vi "GOLPI full test.vi"() -> ()   [LabVIEW 2020, in "GOLPI library.lvlib"]
doc: "Makes test of all routines in GOLPI library. Good for testing changes in GOLPI library or testing compatibility with new versions of GNU Octave."
uses:
  GOLPI library.lvlib
  Type Definitions/Transfer Mode.ctl
  Type Definitions/Custom Error Codes Enum Type Def.vi
  Set Variable - polymorph parts/Set Double.vi
  Get Variable - polymorph parts/Get Double.vi
  Set Variable - polymorph parts/Set Double Complex.vi
  Get Variable - polymorph parts/Get Double Complex.vi
  Set Variable - polymorph parts/Set 2D Array Double.vi
  Get Variable - polymorph parts/Get 2D Array Double.vi
  Set Variable - polymorph parts/Set 2D Array Double Complex.vi
  Get Variable - polymorph parts/Get 2D Array Double Complex.vi
  Set Variable - polymorph parts/Set String.vi
  Get Variable - polymorph parts/Get String.vi
  Set Variable - polymorph parts/Set 1D Array String.vi
  Get Variable - polymorph parts/Get 1D Array String.vi
panel:
  out "file (write)":dbl format="%#_3p"
  out "pipe (write)":dbl format="%#_3p"
  out "console (write)":dbl format="%#_3p"
  out "pipe":dbl format="%#_3p"
  out "bitstream":dbl format="%#_3p"
  out "State":string
  in  "skip read to ...\n tests?":bool
  out "mode":T1
  in  "Matlab\nmode":bool
  out "file":dbl format="%#_3p"
  out "console":dbl format="%#_3p"
  in  "wait for exit\n(press this again to exit)":bool
  in  "hide window":bool
  out "now running test no:":i32
  out "all tests result":bool
  out "test results":T2(array[cluster])
  in  "do tests with large\nrandom datasets?":bool
  out "GNU Octave version":string
  out "exit code":i32
  out "error out":errorcluster
  in  "Octave binary directory":path=path "C:/Octave/Octave-4.2.2/bin/octave-cli.exe"
  in  "Working directory":path=path "C:/work"
  # "Runs various tests and checks all parts of GOLPI library.\nSelecting 'do tests with large random datasets' cause\nrunning of time consuming tests.\nIf all tests are OK, GOLPI is fully working with selected\nGNU Octave binary.\nIF WORKING DIRECTORY IS NOT WRITEABLE (C:\\ in Win7+), tests will fail also."
  # "Time consumed reading/writting large random matrix (s) using:"
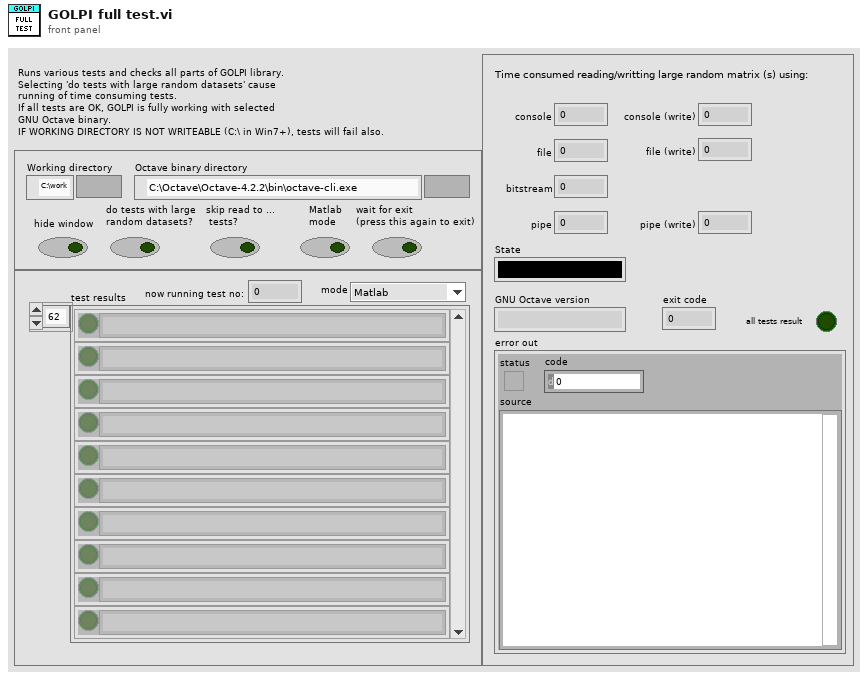
[diagram p1: front panel]
types:
  T1 = typedef "GOLPI library.lvlib/Transfer Mode.ctl" = enum16{"Matlab", "stdio", "temp file", "bitstream", "pipe"}
  T2 = cluster{"test result":bool, "variable name":string}[]
  T3 = typedef "GOLPI library.lvlib/GOLPI reference Type Def.ctl" = cluster{"pipe handle":T4, "fast read timeout [ms]":u32, "fast read settle time [ms]":u32, "fast read to multiple [ms]":u32, "max elements per input line":u32, "slow read timeout [ms]":u32, "stdin double format specifier":string, "max elements per stdout output column":u32, "console mode bitstream":bool, "bitstream first read timeout [ms]":u32, "bitstream read timeout [ms]":u32, "struct transfer possible":bool, "matlab mode":bool, "var pipe write timeout [ms]":u32, "variable pipe mode":bool, "variable pipe buffer size [Bytes]":u32, "variable pipe block size [Bytes]":u32}
  T4 = typedef "LV Process library.lvlib/Pipe Handle.ctl" = cluster{"lv_proc.dll file path":path, "process instance handle":u32[], "debug mode":bool, "debug data":cluster{"time":timestamp, "stdin":bool, "data":string}[]}
  T5 = typedef "GOLPI library.lvlib/Custom Error Codes Enum Type Def.vi" = enum16{"no error", "00 working directory PAR1 missing", "01 octave binary PAR1 missing", "02 octave report error PAR1", "03 empty output last cmd PAR1", "04 missing temporary file PAR1", "05 pwd PAR 1 not exist", "06 oct package not installed", "07 octave default binary missing", "10 var PAR1 not string, vect", "11 var PAR1 not num, scal, ~compl", "12 var PAR1 not num, scal, compl", "13 var PAR1 not num, vect, ~compl", "14 var PAR1 not num, vect, compl", "15 var PAR1 not num, mat, ~compl", "16 var PAR1 not num, mat, ~compl", "30 read timeout", "60 bitstream transport failed", "61 bitstream decode error PAR1", "62 bitstream cannot be set", "70 struct transfer not possible", "80 struct: cluster elem. PAR1 not implem.", "81 struct: structure field PAR1 not implem.", "82 struct: size mismatch of PAR1", "83 struct: type mismatch of PAR1", "98 internal error", "99 not finished", "90 Not supported in Matlab mode", "91 Matlab variable transfer error", "92 Matlab Script Error", "100 Variable Pipe Mode cannot be set"}
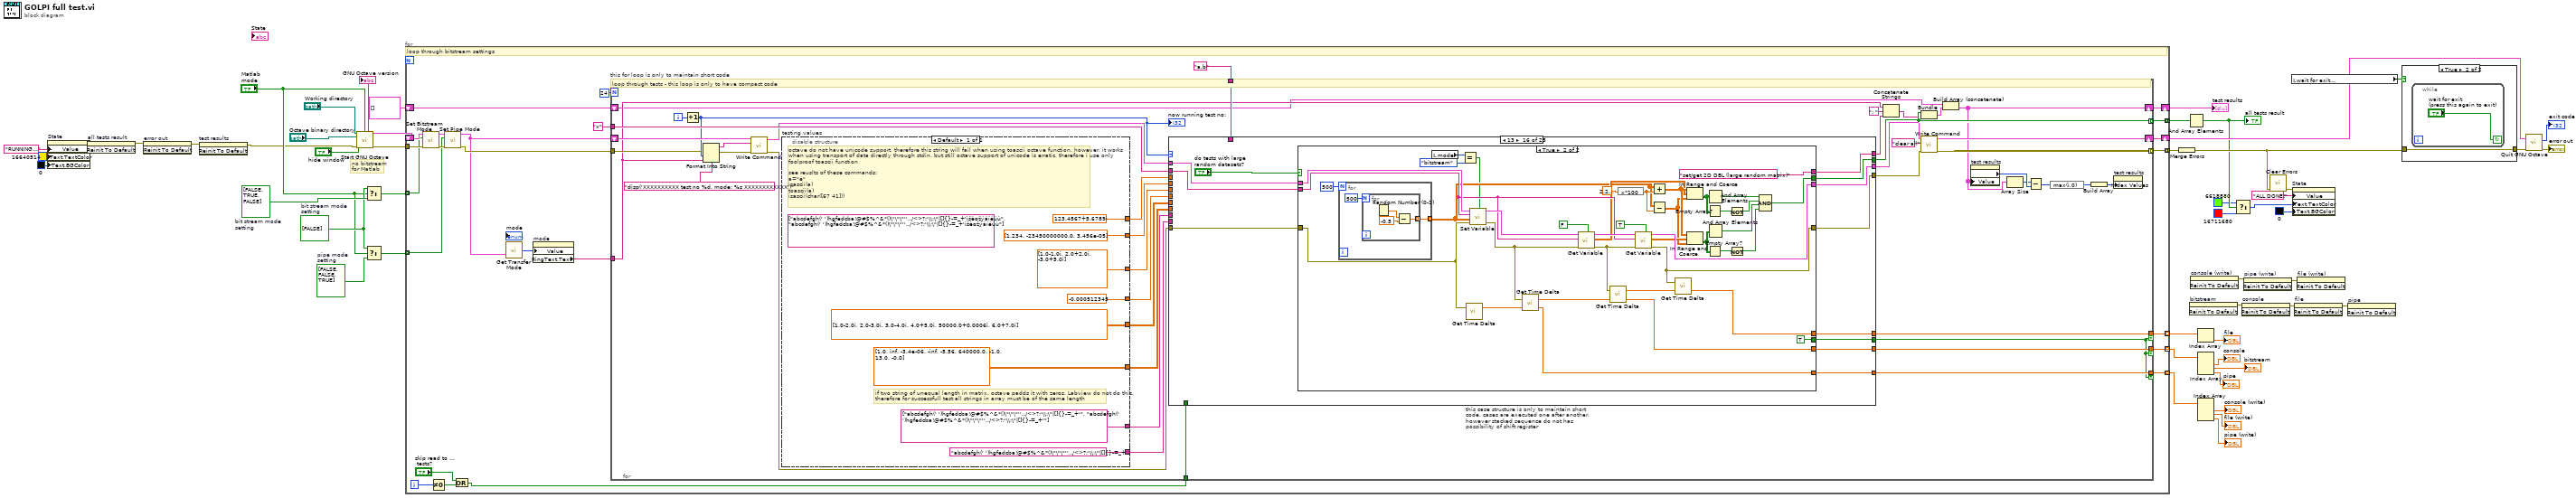
[diagram p0: block diagram]
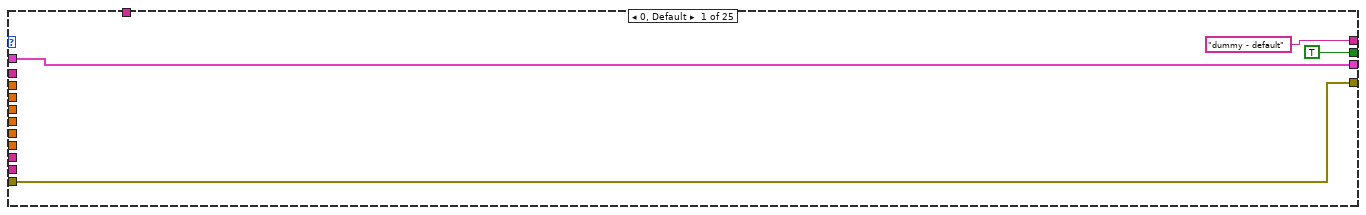
[diagram p3: hidden frame]
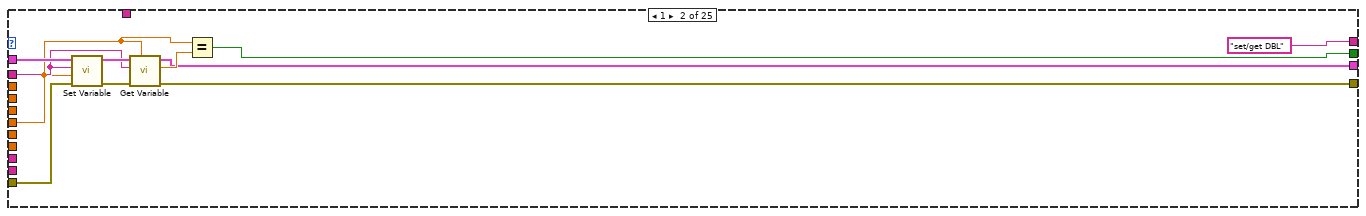
[diagram p4: hidden frame]
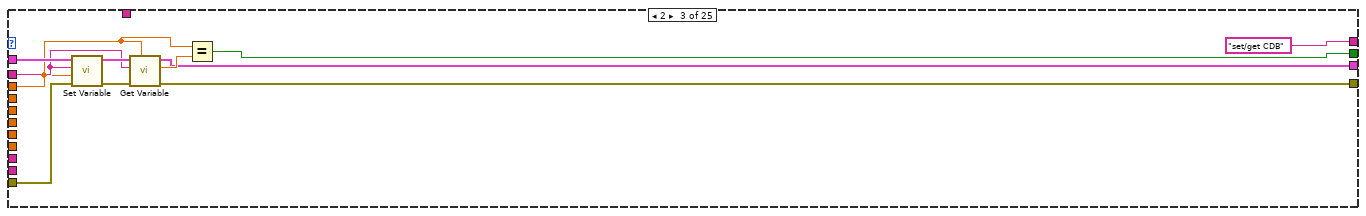
[diagram p5: hidden frame]
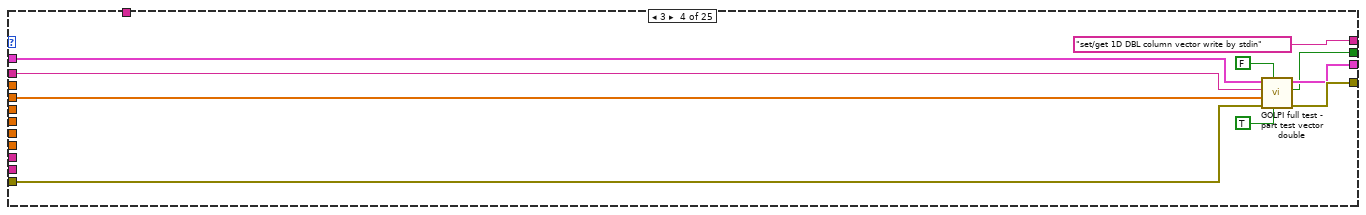
[diagram p6: hidden frame]
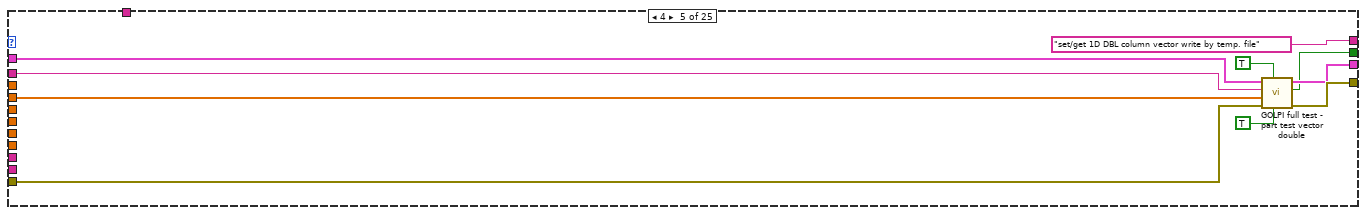
[diagram p7: hidden frame]
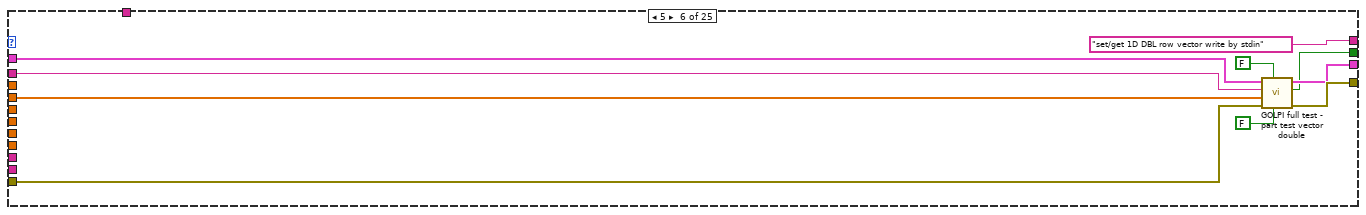
[diagram p8: hidden frame]
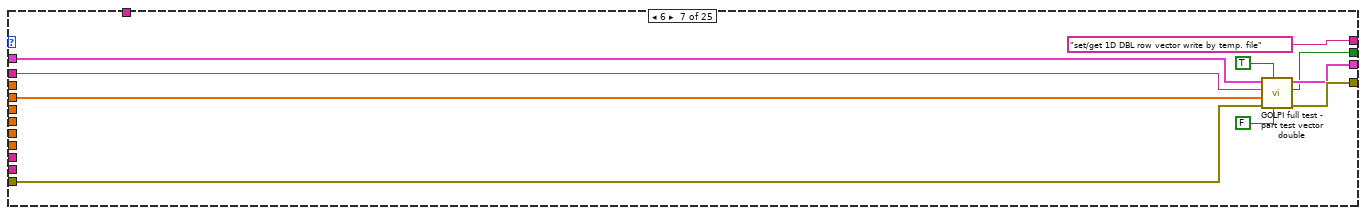
[diagram p9: hidden frame]
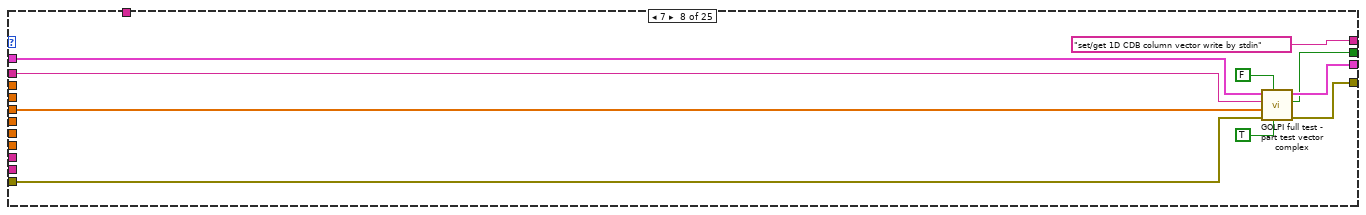
[diagram p10: hidden frame]
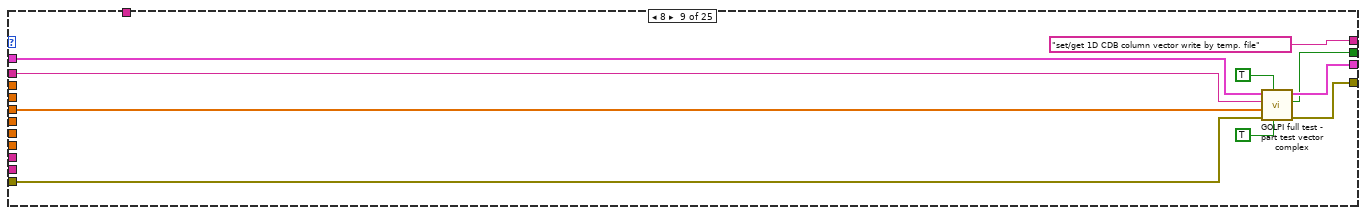
[diagram p11: hidden frame]
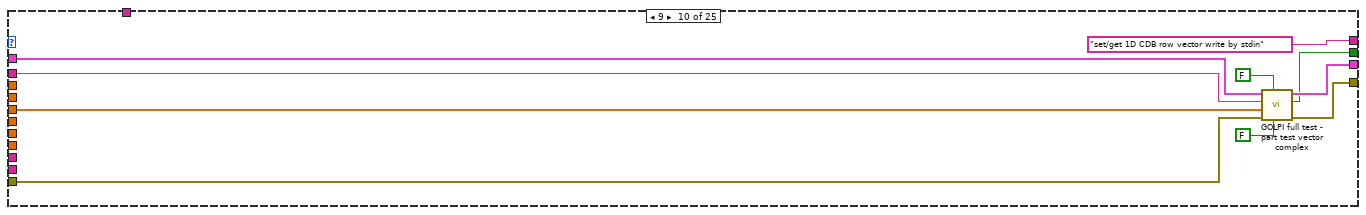
[diagram p12: hidden frame]
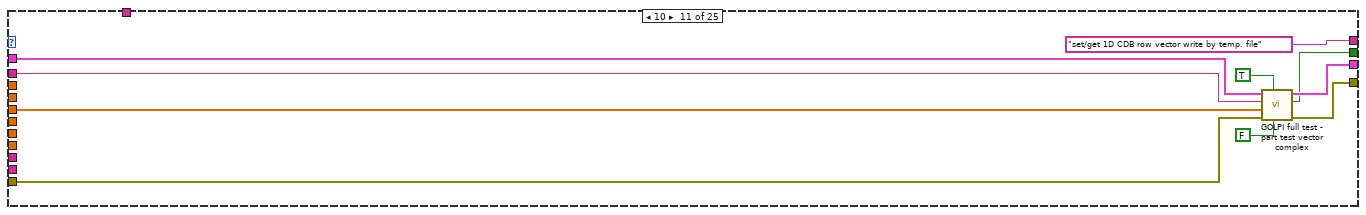
[diagram p13: hidden frame]
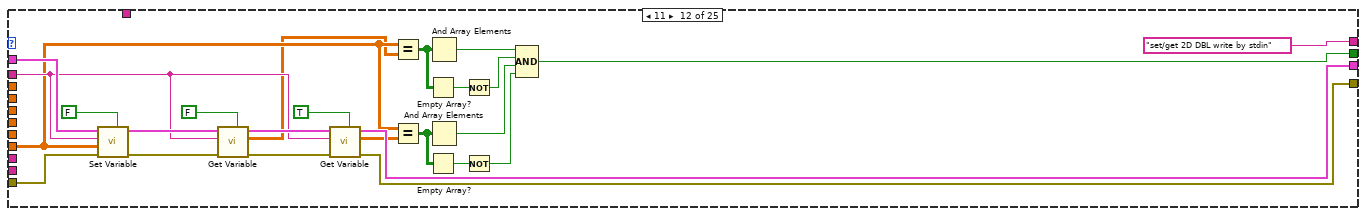
[diagram p14: hidden frame]
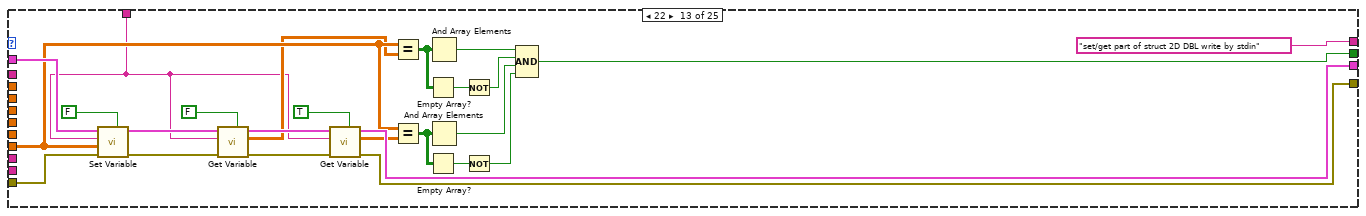
[diagram p15: hidden frame]
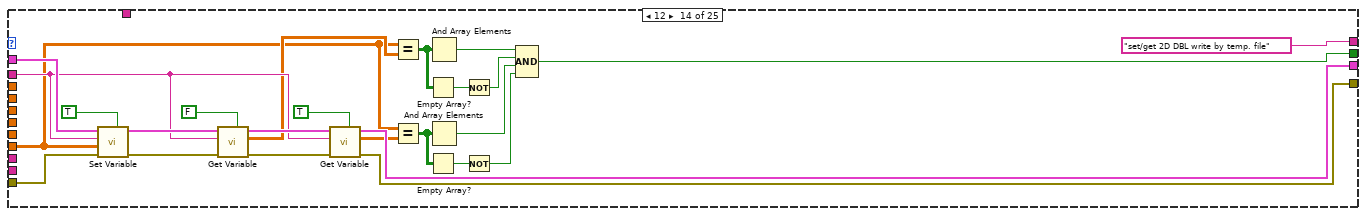
[diagram p16: hidden frame]
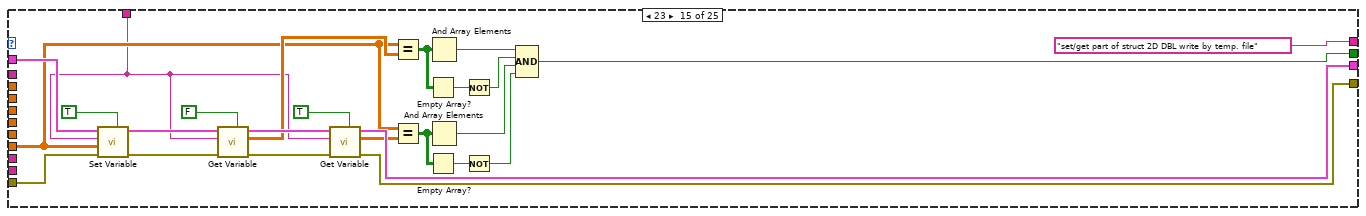
[diagram p17: hidden frame]
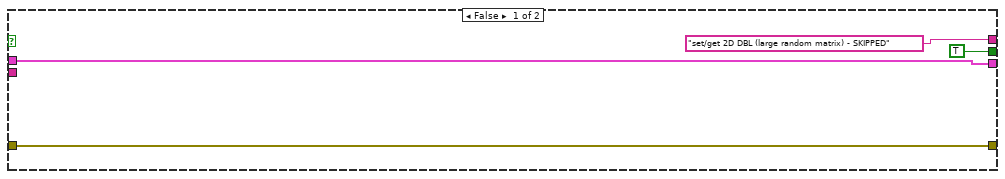
[diagram p18: hidden frame]
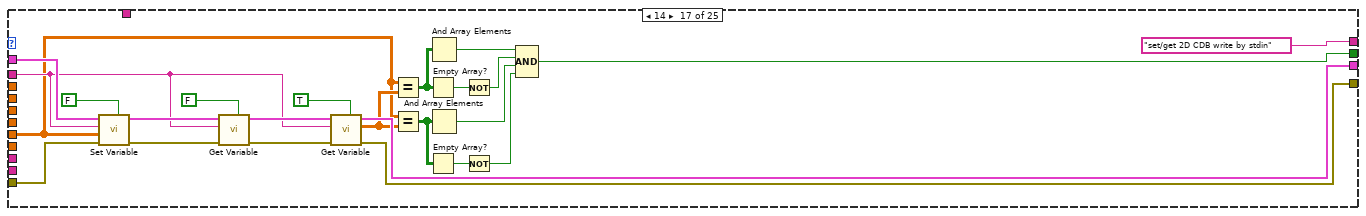
[diagram p19: hidden frame]
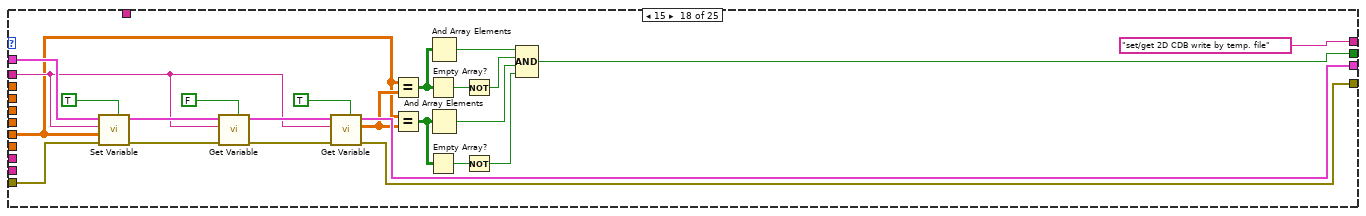
[diagram p20: hidden frame]
diagram:
  w38 = bool[] [FALSE, FALSE, TRUE]  # pipe mode setting
  w39 = bool[] [FALSE]  # bit stream mode setting
  w41 = bool[] [FALSE, TRUE, FALSE]  # bit stream mode setting
  # "no bitstream\nfor Matlab"
  n1 = property on="State" class="Str"("Value"="RUNNING..." ("State"), "Text.TextColor"=u32 16640514 ("Text.Text Colors:Text Color"), "Text.BGColor"=u32 0 ("Text.Text Colors:BG Color")) -> (error out=w27:errorcluster)  [unwired: 2 in, 1 out]
  n2 = invoke on="all tests result" class="Bool (strict)" method="Reinit To Default"(error in=w27) -> (error out=w28:errorcluster)  [unwired: 2 in, 2 out]
  n3 = invoke on="error out" class="Clust (strict)" method="Reinit To Default"(error in=w28) -> (error out=w36:errorcluster)  [unwired: 2 in, 2 out]
  n4 = invoke on="test results" class="Arr (strict)" method="Reinit To Default"(error in=w36) -> (error out=w35:errorcluster)  [unwired: 2 in, 2 out]
  n5 = call "Start GNU Octave.vi"("working dir (user home)"="Working directory", "Matlab script mode (F)"="Matlab\nmode", "octave binary file or dir (autofind)"="Octave binary directory", "hide debug console (T)"="hide window", "error in"=w35) -> ("GNU Octave version"=→"GNU Octave version":string, "GOLPI ref. out"=w45:T3, "error out"=w49:errorcluster)  [unwired: 7 in, 1 out]
  n6 = Select(t=w39, s="Matlab\nmode", f=w41) -> (s? t:f=w42:bool[])
  n7 = Select(t=w39, s="Matlab\nmode", f=w38) -> (s? t:f=w40:bool[])
  n8 = for {
    tunnel: [w73] -> w48 mode=concatenating
    shift-right: [w75] -> w43
    shift-left: w45 -> [w69]
    tunnel: w42 -> [w68] mode=indexing
    tunnel: w49 -> [w70]
    tunnel: [w71] -> w44 mode=concatenating
    tunnel: w40 -> [w64] mode=indexing
    shift-right: [w56] -> w30
    shift-left: cluster{"test result":bool, string}[] [] -> [w55]
    tunnel: [w54] -> w15 mode=indexing
    tunnel: [w53] -> w13 mode=indexing
    tunnel: [w52] -> w6 mode=indexing
    i -> [w60]
    # "loop through bitstream settings"
    n9 = call "Set Bitstream Mode.vi"("error in"=w70, "Bitstream mode (F)"=w68, "GOLPI ref. in"=w69) -> ("error out"=w67:errorcluster, "GOLPI ref. out"=w66:T3)  [unwired: 7 in]
    n10 = Not Equal To 0?(x=w60) -> (x != 0?=w59:bool)
    n11 = call "Set Pipe Mode.vi"("error in"=w67, "Variable Pipe Mode? (F)"=w64, "GOLPI ref. in"=w66) -> ("error out"=w65:errorcluster, "GOLPI ref. out"=w63:T3)  [unwired: 7 in]
    n12 = Compound Arithmetic op=OR("skip read to ...\n tests?", w59) -> (w57:bool)
    n13 = call "Get Transfer Mode.vi"("GOLPI ref."=w63) -> ("mode"=w62:T1)  [unwired: 1 in]
    n14 = property on="mode" class="Enum (strict)"("Value"=w62) -> ("RingText.Text"=w61:string)  [unwired: 2 in, 2 out]
    n15 = for "this for loop is only to maintain short code" {
      N: 24 -> [_]
      tunnel: "x" ("variable name") -> [w118]
      shift-right: [w114] -> w75
      shift-left: w63 -> [w100]
      tunnel: [w116] -> w73 mode=indexing
      tunnel: "a.b" ("variable name") -> [w102]
      tunnel: w65 -> [w96]
      tunnel: [w112] -> w71 mode=indexing
      tunnel: w61 -> [w91]
      tunnel: w57 -> [w89]
      shift-right: [w81] -> w56
      shift-left: w55 -> [w87]
      tunnel: [w80] -> w54 if=w77
      tunnel: [w79] -> w53 if=w77
      tunnel: [w78] -> w52 if=w77
      i -> [w117]
      # "loop through tests - this loop is only to have compact code"
      n16 = Increment(x=w117) -> (x+1=w97:i32)
      "now running test no:" <- w97
      n17 = Format Into String(format string="disp('XXXXXXXXXX test no %d, mode: %s XXXXXXXXXXXX')", error in=w96, w97, w91) -> (resulting string=w94:string, error out=w95:errorcluster)  [unwired: 1 in]
      n18 = call "Write Command.vi"("error in"=w95, "command"=w94, "GOLPI ref. in"=w100) -> ("error out"=w101:errorcluster, "GOLPI ref. out"=w99:T3)  [unwired: 7 in]
      n19 = disable-structure "testing values" shown="Default" {
        disable-tunnel: [-0.000512345 ("value")] -> w110
        disable-tunnel: [dbl[] [1.234, -23450000000.0, 3.456e-05] ("value")] -> w109
        disable-tunnel: [cdb[] [1.0-1.0i, 2.0+2.0i, -3.0+5.0i] ("value")] -> w108
        disable-tunnel: [dbl[][] [[1.0, inf, -3.4e-06], [-inf, -5.56, 640000.0], [-1.0, 13.0, -0.0]] ("value")] -> w107
        disable-tunnel: [cdb[][] [[1.0-2.0i, 2.0-3.0i, 3.0-4.0i], [4.0+5.0i, 50000.0+0.0006i, 6.0+7.0i]] ("value")] -> w106
        disable-tunnel: ["abcdefgh(' ')hgfedcba!@#$%^&*()\"\"\"'',./<>?;'\\:\"|[]{}-=_+'" ("value")] -> w105
        disable-tunnel: [string[] ["abcdefgh(' ')hgfedcba!@#$%^&*()\"\"\"'',./<>?;'\\:\"|[]{}-=_+'", "abcdefgh(' ')hgfedcba!@#$%^&*()\"\"\"'',./<>?;'\\:\"|[]{}-=_+'"]] -> w104
        disable-tunnel: [cdb 123.4567+5.6789i ("value")] -> w103
        frame Enabled {
          (unwired) string[] ["abcdefgh(' ')hgfedcba!@#$%^&*()\"\"\"'',./<>?;'\\:\"|[]{}-=_+'ìšèøžýáíéúù", "abcdefgh(' ')hgfedcba!@#$%^&*()\"\"\"'',./<>?;'\\:\"|[]{}-=_+'ìšèøžýáíéúù"]
          # "octave do not have unicode support, therefore this string will fail when using toascii octave function. however, it works\nwhen using transport of data directly through stdin. but still octave support of unicode is erratic, therefore i use only\nfoolproof toascii function\n\nsee reuslts of these commands:\na=\"é\"\nisascii(a)\ntoascii(a)\nisascii(char([67 41]))"
          # "if two string of unequal length in matrix, octave padds it with zeros. Labview do not do this.\ntherefore for successfull test all strings in array must be of the same length"
        }
      }
      n20 = case "this case structure is only to maintain short code. cases are executed one after another. however stacked sequence do not has possibility of shift register" shown="13" w97 {
        tunnel: w99 -> [w129 w138 w145 w158 w168 w180 w190 w202 w212 w219 w229 w253 w278 w303 w328 w340 w415 w439 w457 w476 w501 w526 w535 w565 w600]
        tunnel: w101 -> [w130 w137 w146 w161 w171 w182 w192 w199 w209 w222 w232 w254 w279 w304 w329 w341 w416 w440 w458 w477 w502 w527 w534 w564 w601]
        tunnel: [w130 w136 w147 w160 w170 w179 w189 w200 w210 w221 w231 w256 w281 w306 w331 w343 w414 w438 w450 w467 w489 w510 w531 w560 w593] -> w113
        tunnel: [w129 w135 w148 w159 w169 w178 w188 w201 w211 w220 w230 w255 w280 w305 w330 w342 w413 w437 w451 w465 w488 w512 w533 w562 w599] -> w115
        tunnel: w118 -> [_ w134 w144 w157 w167 w181 w191 w198 w208 w218 w228 w240 _ w290 _ w339 w395 w419 w448 w461 w487 w509 _ _ _]
        tunnel: [TRUE w133 w149 w154 w164 w177 w187 w196 w206 w215 w225 w257 w282 w307 w332 w344 w412 w436 w442 w463 w492 w517 w532 w561 w591] -> w116
        tunnel: ["dummy - default" ("variable name") "set/get DBL" ("variable name") "set/get CDB" ("variable name") "set/get 1D DBL column vector write by stdin" ("variable name") "set/get 1D DBL column vector write by temp. file" ("variable name") "set/get 1D DBL row vector write by stdin" ("variable name") "set/get 1D DBL row vector write by temp. file" ("variable name") "set/get 1D CDB column vector write by stdin" ("variable name") "set/get 1D CDB column vector write by temp. file" ("variable name") "set/get 1D CDB row vector write by stdin" ("variable name") "set/get 1D CDB row vector write by temp. file" ("variable name") "set/get 2D DBL write by stdin" ("variable name") "set/get part of struct 2D DBL write by stdin" ("variable name") "set/get 2D DBL write by temp. file" ("variable name") "set/get part of struct 2D DBL write by temp. file" ("variable name") w338 "set/get 2D CDB write by stdin" ("variable name") "set/get 2D CDB write by temp. file" ("variable name") "set/get STR write by stdin" ("variable name") "set/get STR write by temp. file" ("variable name") "set/get 1D STR write by stdin" ("variable name") "set/get 1D STR write by temp. file" ("variable name") w530 w563 "read struct" ("variable name")] -> w93
        tunnel: w110 -> [_ w131 _ _ _ _ _ _ _ _ _ _ _ _ _ _ _ _ _ _ _ _ _ _ _]
        tunnel: w103 -> [_ _ w142 _ _ _ _ _ _ _ _ _ _ _ _ _ _ _ _ _ _ _ _ _ _]
        tunnel: w109 -> [_ _ _ w153 w163 w173 w183 _ _ _ _ _ _ _ _ _ _ _ _ _ _ _ _ _ _]
        tunnel: w108 -> [_ _ _ _ _ _ _ w193 w203 w213 w223 _ _ _ _ _ _ _ _ _ _ _ _ _ _]
        tunnel: w107 -> [_ _ _ _ _ _ _ _ _ _ _ w235 w261 w283 w309 _ _ _ _ _ _ _ _ _ _]
        tunnel: w106 -> [_ _ _ _ _ _ _ _ _ _ _ _ _ _ _ _ w393 w417 _ _ _ _ _ _ _]
        tunnel: w105 -> [_ _ _ _ _ _ _ _ _ _ _ _ _ _ _ _ _ _ w441 w460 _ _ _ _ _]
        tunnel: w104 -> [_ _ _ _ _ _ _ _ _ _ _ _ _ _ _ _ _ _ _ _ w479 w504 _ _ _]
        tunnel: w102 -> [_ _ _ _ _ _ _ _ _ _ _ _ w258 _ w308 _ _ _ _ _ _ _ _ _ _]
        tunnel: w89 -> [_ _ _ _ _ _ _ _ _ _ _ _ _ _ _ _ _ _ _ _ _ _ w529 w559 _]
        tunnel: [_ _ _ _ _ _ _ _ _ _ _ _ _ _ _ w336 _ _ _ _ _ _ _ _ _] -> w80
        tunnel: [_ _ _ _ _ _ _ _ _ _ _ _ _ _ _ w335 _ _ _ _ _ _ _ _ _] -> w79
        tunnel: [_ _ _ _ _ _ _ _ _ _ _ _ _ _ _ w334 _ _ _ _ _ _ _ _ _] -> w77
        tunnel: [_ _ _ _ _ _ _ _ _ _ _ _ _ _ _ w333 _ _ _ _ _ _ _ _ _] -> w78
        frame 0, Default {
        }
        frame 1 {
          n21 = call-poly "Set Variable.vi"("error in"=w137, "value"=w131, "variable name"=w134, "GOLPI ref. in"=w138) -> ("error out"=w140:errorcluster, "GOLPI ref. out"=w141:T3)  [unwired: 6 in]
          n22 = call-poly "Get Variable.vi"("data type of variable"=w131, "error in"=w140, "variable name"=w134, "GOLPI ref. in"=w141) -> ("error out"=w136:errorcluster, "value"=w139:dbl, "GOLPI ref. out"=w135:T3)  [unwired: 5 in]
          n23 = Equal?(x=w131, y=w139) -> (x = y?=w133:bool)
        }
        frame 2 {
          n24 = call-poly "Set Variable.vi"("error in"=w146, "value"=w142, "variable name"=w144, "GOLPI ref. in"=w145) -> ("error out"=w151:errorcluster, "GOLPI ref. out"=w150:T3)  [unwired: 6 in]
          n25 = call-poly "Get Variable.vi"("data type of variable"=w142, "error in"=w151, "variable name"=w144, "GOLPI ref. in"=w150) -> ("error out"=w147:errorcluster, "value"=w152:cdb, "GOLPI ref. out"=w148:T3)  [unwired: 5 in]
          n26 = Equal?(x=w142, y=w152) -> (x = y?=w149:bool)
        }
        frame 3 {
          n27 = call "GOLPI full test - part test vector double.vi"("column vector?"=TRUE, "set: use temporary file?"=FALSE, "error in (no error)"=w161, "test value"=w153, "variable name in"=w157, "GOLPI ref. in"=w158) -> ("error out"=w160:errorcluster, "test result"=w154:bool, "GOLPI ref. out"=w159:T3)  [unwired: 3 in]
        }
        frame 4 {
          n28 = call "GOLPI full test - part test vector double.vi"("column vector?"=TRUE, "set: use temporary file?"=TRUE, "error in (no error)"=w171, "test value"=w163, "variable name in"=w167, "GOLPI ref. in"=w168) -> ("error out"=w170:errorcluster, "test result"=w164:bool, "GOLPI ref. out"=w169:T3)  [unwired: 3 in]
        }
        frame 5 {
          n29 = call "GOLPI full test - part test vector double.vi"("column vector?"=FALSE, "set: use temporary file?"=FALSE, "error in (no error)"=w182, "test value"=w173, "variable name in"=w181, "GOLPI ref. in"=w180) -> ("error out"=w179:errorcluster, "test result"=w177:bool, "GOLPI ref. out"=w178:T3)  [unwired: 3 in]
        }
        frame 6 {
          n30 = call "GOLPI full test - part test vector double.vi"("column vector?"=FALSE, "set: use temporary file?"=TRUE, "error in (no error)"=w192, "test value"=w183, "variable name in"=w191, "GOLPI ref. in"=w190) -> ("error out"=w189:errorcluster, "test result"=w187:bool, "GOLPI ref. out"=w188:T3)  [unwired: 3 in]
        }
        frame 7 {
          n31 = call "GOLPI full test - part test vector complex.vi"("column vector?"=TRUE, "set: use temporary file?"=FALSE, "error in (no error)"=w199, "test value"=w193, "variable name in"=w198, "GOLPI ref. in"=w202) -> ("error out"=w200:errorcluster, "test result"=w196:bool, "GOLPI ref. out"=w201:T3)  [unwired: 3 in]
        }
        frame 8 {
          n32 = call "GOLPI full test - part test vector complex.vi"("column vector?"=TRUE, "set: use temporary file?"=TRUE, "error in (no error)"=w209, "test value"=w203, "variable name in"=w208, "GOLPI ref. in"=w212) -> ("error out"=w210:errorcluster, "test result"=w206:bool, "GOLPI ref. out"=w211:T3)  [unwired: 3 in]
        }
        frame 9 {
          n33 = call "GOLPI full test - part test vector complex.vi"("column vector?"=FALSE, "set: use temporary file?"=FALSE, "error in (no error)"=w222, "test value"=w213, "variable name in"=w218, "GOLPI ref. in"=w219) -> ("error out"=w221:errorcluster, "test result"=w215:bool, "GOLPI ref. out"=w220:T3)  [unwired: 3 in]
        }
        frame 10 {
          n34 = call "GOLPI full test - part test vector complex.vi"("column vector?"=FALSE, "set: use temporary file?"=TRUE, "error in (no error)"=w232, "test value"=w223, "variable name in"=w228, "GOLPI ref. in"=w229) -> ("error out"=w231:errorcluster, "test result"=w225:bool, "GOLPI ref. out"=w230:T3)  [unwired: 3 in]
        }
        frame 11 {
          n35 = call-poly "Set Variable.vi"("use temporary file? (F)"=FALSE ("use temporary file?"), "error in"=w254, "value"=w235, "variable name"=w240, "GOLPI ref. in"=w253) -> ("error out"=w244:errorcluster, "GOLPI ref. out"=w242:T3)  [unwired: 5 in]
          n36 = call-poly "Get Variable.vi"("use temporary file? (F)"=FALSE ("use temporary file?"), "error in"=w244, "variable name"=w240, "GOLPI ref. in"=w242) -> ("error out"=w243:errorcluster, "value"=w234:dbl[][], "GOLPI ref. out"=w241:T3)  [unwired: 5 in]
          n37 = call-poly "Get Variable.vi"("use temporary file? (F)"=TRUE ("use temporary file?"), "error in"=w243, "variable name"=w240, "GOLPI ref. in"=w241) -> ("error out"=w256:errorcluster, "value"=w246:dbl[][], "GOLPI ref. out"=w255:T3)  [unwired: 5 in]
          n38 = Equal?(x=w235, y=w234) -> (x = y?=w233:bool[][])
          n39 = Equal?(x=w235, y=w246) -> (x = y?=w248:bool[][])
          n40 = Empty Array?(array=w233) -> (empty?=w238:bool)
          n41 = Empty Array?(array=w248) -> (empty?=w249:bool)
          n42 = And Array Elements(Boolean array=w233) -> (logical AND=w239:bool)
          n43 = And Array Elements(Boolean array=w248) -> (logical AND=w251:bool)
          n44 = Not(x=w238) -> (.not. x?=w237:bool)
          n45 = Not(x=w249) -> (.not. x?=w250:bool)
          n46 = Compound Arithmetic op=AND(w239, w237, w251, w250) -> (w257:bool)
        }
        frame 22 {
          n47 = call-poly "Set Variable.vi"("use temporary file? (F)"=FALSE ("use temporary file?"), "error in"=w279, "value"=w261, "variable name"=w258, "GOLPI ref. in"=w278) -> ("error out"=w269:errorcluster, "GOLPI ref. out"=w267:T3)  [unwired: 5 in]
          n48 = call-poly "Get Variable.vi"("use temporary file? (F)"=FALSE ("use temporary file?"), "error in"=w269, "variable name"=w258, "GOLPI ref. in"=w267) -> ("error out"=w268:errorcluster, "value"=w260:dbl[][], "GOLPI ref. out"=w266:T3)  [unwired: 5 in]
          n49 = call-poly "Get Variable.vi"("use temporary file? (F)"=TRUE ("use temporary file?"), "error in"=w268, "variable name"=w258, "GOLPI ref. in"=w266) -> ("error out"=w281:errorcluster, "value"=w271:dbl[][], "GOLPI ref. out"=w280:T3)  [unwired: 5 in]
          n50 = Equal?(x=w261, y=w260) -> (x = y?=w259:bool[][])
          n51 = Equal?(x=w261, y=w271) -> (x = y?=w273:bool[][])
          n52 = Empty Array?(array=w259) -> (empty?=w264:bool)
          n53 = Empty Array?(array=w273) -> (empty?=w274:bool)
          n54 = And Array Elements(Boolean array=w259) -> (logical AND=w265:bool)
          n55 = And Array Elements(Boolean array=w273) -> (logical AND=w276:bool)
          n56 = Not(x=w264) -> (.not. x?=w263:bool)
          n57 = Not(x=w274) -> (.not. x?=w275:bool)
          n58 = Compound Arithmetic op=AND(w265, w263, w276, w275) -> (w282:bool)
        }
        frame 12 {
          n59 = call-poly "Set Variable.vi"("use temporary file? (F)"=TRUE ("use temporary file?"), "error in"=w304, "value"=w283, "variable name"=w290, "GOLPI ref. in"=w303) -> ("error out"=w294:errorcluster, "GOLPI ref. out"=w292:T3)  [unwired: 5 in]
          n60 = call-poly "Get Variable.vi"("use temporary file? (F)"=FALSE ("use temporary file?"), "error in"=w294, "variable name"=w290, "GOLPI ref. in"=w292) -> ("error out"=w293:errorcluster, "value"=w288:dbl[][], "GOLPI ref. out"=w291:T3)  [unwired: 5 in]
          n61 = call-poly "Get Variable.vi"("use temporary file? (F)"=TRUE ("use temporary file?"), "error in"=w293, "variable name"=w290, "GOLPI ref. in"=w291) -> ("error out"=w306:errorcluster, "value"=w296:dbl[][], "GOLPI ref. out"=w305:T3)  [unwired: 5 in]
          n62 = Equal?(x=w283, y=w288) -> (x = y?=w289:bool[][])
          n63 = Equal?(x=w283, y=w296) -> (x = y?=w298:bool[][])
          n64 = Empty Array?(array=w289) -> (empty?=w286:bool)
          n65 = Empty Array?(array=w298) -> (empty?=w299:bool)
          n66 = And Array Elements(Boolean array=w289) -> (logical AND=w287:bool)
          n67 = And Array Elements(Boolean array=w298) -> (logical AND=w301:bool)
          n68 = Not(x=w286) -> (.not. x?=w285:bool)
          n69 = Not(x=w299) -> (.not. x?=w300:bool)
          n70 = Compound Arithmetic op=AND(w287, w285, w301, w300) -> (w307:bool)
        }
        frame 23 {
          n71 = call-poly "Set Variable.vi"("use temporary file? (F)"=TRUE ("use temporary file?"), "error in"=w329, "value"=w309, "variable name"=w308, "GOLPI ref. in"=w328) -> ("error out"=w319:errorcluster, "GOLPI ref. out"=w317:T3)  [unwired: 5 in]
          n72 = call-poly "Get Variable.vi"("use temporary file? (F)"=FALSE ("use temporary file?"), "error in"=w319, "variable name"=w308, "GOLPI ref. in"=w317) -> ("error out"=w318:errorcluster, "value"=w314:dbl[][], "GOLPI ref. out"=w316:T3)  [unwired: 5 in]
          n73 = call-poly "Get Variable.vi"("use temporary file? (F)"=TRUE ("use temporary file?"), "error in"=w318, "variable name"=w308, "GOLPI ref. in"=w316) -> ("error out"=w331:errorcluster, "value"=w321:dbl[][], "GOLPI ref. out"=w330:T3)  [unwired: 5 in]
          n74 = Equal?(x=w309, y=w314) -> (x = y?=w315:bool[][])
          n75 = Equal?(x=w309, y=w321) -> (x = y?=w323:bool[][])
          n76 = Empty Array?(array=w315) -> (empty?=w312:bool)
          n77 = Empty Array?(array=w323) -> (empty?=w324:bool)
          n78 = And Array Elements(Boolean array=w315) -> (logical AND=w313:bool)
          n79 = And Array Elements(Boolean array=w323) -> (logical AND=w326:bool)
          n80 = Not(x=w312) -> (.not. x?=w311:bool)
          n81 = Not(x=w324) -> (.not. x?=w325:bool)
          n82 = Compound Arithmetic op=AND(w313, w311, w326, w325) -> (w332:bool)
        }
        frame 13 {
          n83 = case shown="True" "do tests with large\nrandom datasets?" {
            tunnel: [TRUE w383] -> w344
            tunnel: [w348 w358] -> w343
            tunnel: [w347 w382] -> w342
            tunnel: w341 -> [w348 w354]
            tunnel: w340 -> [w347 w381]
            tunnel: w339 -> [_ w369]
            tunnel: ["set/get 2D DBL (large random matrix) - SKIPPED" ("variable name") "set/get 2D DBL (large random matrix)" ("variable name")] -> w338
            tunnel: [_ w356] -> w336
            tunnel: [_ w355] -> w335
            tunnel: [_ TRUE] -> w334
            tunnel: [_ w352] -> w333
            frame False {
            }
            frame True {
              n84 = for {
                N: 500 ("dimension size") -> [_]
                tunnel: [w389] -> w363 mode=indexing
                n85 = for {
                  N: 500 ("dimension size") -> [_]
                  tunnel: [w390] -> w389 mode=indexing
                  n86 = Random Number (0-1)() -> (number: 0 to 1=w392:dbl)
                  n87 = Subtract(x=w392, y=-0.5) -> (x-y=w390:dbl)
                }
              }
              n88 = local read "mode"() -> (w351:T1)
              n89 = Equal?(x=w351, y=Transfer_Mode."bitstream") -> (x = y?=w349:bool)
              n90 = call "Get Time Delta.vi"("anything in (for synchronization)"=w354) -> ("time now"=w353:dbl)  [unwired: 1 in, 1 out]
              n91 = call-poly "Set Variable.vi"("use temporary file? (F)"=w349, "error in"=w354, "value"=w363, "variable name"=w369, "GOLPI ref. in"=w381) -> ("error out"=w361:errorcluster, "GOLPI ref. out"=w376:T3)  [unwired: 5 in]
              n92 = call "Get Time Delta.vi"("reference time (0)"=w353, "anything in (for synchronization)"=w361) -> ("time delta [s]"=w352:dbl, "time now"=w359:dbl)
              n93 = call-poly "Get Variable.vi"("use temporary file? (F)"=FALSE ("use temporary file?"), "error in"=w361, "variable name"=w369, "GOLPI ref. in"=w376) -> ("error out"=w360:errorcluster, "value"=w368:dbl[][], "GOLPI ref. out"=w375:T3)  [unwired: 5 in]
              n94 = call "Get Time Delta.vi"("reference time (0)"=w359, "anything in (for synchronization)"=w360) -> ("time delta [s]"=w355:dbl, "time now"=w357:dbl)
              n95 = expression code="x*100"(2.220446049250313e-16) -> (w366:dbl)
              n96 = call-poly "Get Variable.vi"("use temporary file? (F)"=TRUE ("use temporary file?"), "error in"=w360, "variable name"=w369, "GOLPI ref. in"=w375) -> ("error out"=w358:errorcluster, "value"=w378:dbl[][], "GOLPI ref. out"=w382:T3)  [unwired: 5 in]
              n97 = Add(x=w363, y=w366) -> (x+y=w373:dbl[][])
              n98 = Subtract(x=w363, y=w366) -> (x-y=w364:dbl[][])
              n99 = call "Get Time Delta.vi"("reference time (0)"=w357, "anything in (for synchronization)"=w358) -> ("time delta [s]"=w356:dbl)  [unwired: 1 out]
              n100 = In Range and Coerce(upper limit=w373, x=w368, lower limit=w364) -> (In Range?=w365:bool[][])  [unwired: 1 out]
              n101 = In Range and Coerce(upper limit=w373, x=w378, lower limit=w364) -> (In Range?=w377:bool[][])  [unwired: 1 out]
              n102 = Empty Array?(array=w365) -> (empty?=w372:bool)
              n103 = Empty Array?(array=w377) -> (empty?=w385:bool)
              n104 = And Array Elements(Boolean array=w365) -> (logical AND=w371:bool)
              n105 = And Array Elements(Boolean array=w377) -> (logical AND=w387:bool)
              n106 = Not(x=w372) -> (.not. x?=w370:bool)
              n107 = Not(x=w385) -> (.not. x?=w386:bool)
              n108 = Compound Arithmetic op=AND(w371, w370, w387, w386) -> (w383:bool)
            }
          }
        }
        frame 14 {
          n109 = call-poly "Set Variable.vi"("use temporary file? (F)"=FALSE ("use temporary file?"), "error in"=w416, "value"=w393, "variable name"=w395, "GOLPI ref. in"=w415) -> ("error out"=w403:errorcluster, "GOLPI ref. out"=w404:T3)  [unwired: 5 in]
          n110 = call-poly "Get Variable.vi"("use temporary file? (F)"=FALSE ("use temporary file?"), "error in"=w403, "variable name"=w395, "GOLPI ref. in"=w404) -> ("error out"=w401:errorcluster, "GOLPI ref. out"=w402:T3)  [unwired: 5 in, 1 out]
          n111 = call-poly "Get Variable.vi"("use temporary file? (F)"=TRUE ("use temporary file?"), "error in"=w401, "variable name"=w395, "GOLPI ref. in"=w402) -> ("error out"=w414:errorcluster, "value"=w396:cdb[][], "GOLPI ref. out"=w413:T3)  [unwired: 5 in]
          n112 = Equal?(x=w393, y=w396) -> (x = y?=w399:bool[][])
          n113 = Equal?(x=w393, y=w396) -> (x = y?=w409:bool[][])
          n114 = Empty Array?(array=w399) -> (empty?=w400:bool)
          n115 = Empty Array?(array=w409) -> (empty?=w408:bool)
          n116 = And Array Elements(Boolean array=w399) -> (logical AND=w398:bool)
          n117 = And Array Elements(Boolean array=w409) -> (logical AND=w406:bool)
          n118 = Not(x=w400) -> (.not. x?=w397:bool)
          n119 = Not(x=w408) -> (.not. x?=w407:bool)
          n120 = Compound Arithmetic op=AND(w398, w397, w406, w407) -> (w412:bool)
        }
        frame 15 {
          n121 = call-poly "Set Variable.vi"("use temporary file? (F)"=TRUE ("use temporary file?"), "error in"=w440, "value"=w417, "variable name"=w419, "GOLPI ref. in"=w439) -> ("error out"=w427:errorcluster, "GOLPI ref. out"=w428:T3)  [unwired: 5 in]
          n122 = call-poly "Get Variable.vi"("use temporary file? (F)"=FALSE ("use temporary file?"), "error in"=w427, "variable name"=w419, "GOLPI ref. in"=w428) -> ("error out"=w425:errorcluster, "GOLPI ref. out"=w426:T3)  [unwired: 5 in, 1 out]
          n123 = call-poly "Get Variable.vi"("use temporary file? (F)"=TRUE ("use temporary file?"), "error in"=w425, "variable name"=w419, "GOLPI ref. in"=w426) -> ("error out"=w438:errorcluster, "value"=w420:cdb[][], "GOLPI ref. out"=w437:T3)  [unwired: 5 in]
          n124 = Equal?(x=w417, y=w420) -> (x = y?=w423:bool[][])
          n125 = Equal?(x=w417, y=w420) -> (x = y?=w433:bool[][])
          n126 = Empty Array?(array=w423) -> (empty?=w424:bool)
          n127 = Empty Array?(array=w433) -> (empty?=w432:bool)
          n128 = And Array Elements(Boolean array=w423) -> (logical AND=w422:bool)
          n129 = And Array Elements(Boolean array=w433) -> (logical AND=w430:bool)
          n130 = Not(x=w424) -> (.not. x?=w421:bool)
          n131 = Not(x=w432) -> (.not. x?=w431:bool)
          n132 = Compound Arithmetic op=AND(w422, w421, w430, w431) -> (w436:bool)
        }
        frame 16 {
          n133 = call-poly "Set Variable.vi"("use temporary file? (F)"=FALSE ("use temporary file?"), "error in"=w458, "value"=w441, "variable name"=w448, "GOLPI ref. in"=w457) -> ("error out"=w459:errorcluster, "GOLPI ref. out"=w456:T3)  [unwired: 5 in]
          n134 = call-poly "Get Variable.vi"("use temporary file? (F)"=FALSE ("use temporary file?"), "error in"=w459, "variable name"=w448, "GOLPI ref. in"=w456) -> ("error out"=w449:errorcluster, "value"=w455:string, "GOLPI ref. out"=w452:T3)  [unwired: 5 in]
          n135 = call-poly "Get Variable.vi"("use temporary file? (F)"=TRUE ("use temporary file?"), "error in"=w449, "variable name"=w448, "GOLPI ref. in"=w452) -> ("error out"=w450:errorcluster, "value"=w445:string, "GOLPI ref. out"=w451:T3)  [unwired: 5 in]
          n136 = Equal?(x=w441, y=w455) -> (x = y?=w443:bool)
          n137 = Equal?(x=w441, y=w445) -> (x = y?=w444:bool)
          n138 = And(x=w443, y=w444) -> (x .and. y?=w442:bool)
        }
        frame 17 {
          n139 = call-poly "Set Variable.vi"("use temporary file? (F)"=TRUE ("use temporary file?"), "error in"=w477, "value"=w460, "variable name"=w461, "GOLPI ref. in"=w476) -> ("error out"=w478:errorcluster, "GOLPI ref. out"=w475:T3)  [unwired: 5 in]
          n140 = call-poly "Get Variable.vi"("use temporary file? (F)"=FALSE ("use temporary file?"), "error in"=w478, "variable name"=w461, "GOLPI ref. in"=w475) -> ("error out"=w468:errorcluster, "value"=w474:string, "GOLPI ref. out"=w466:T3)  [unwired: 5 in]
          n141 = call-poly "Get Variable.vi"("use temporary file? (F)"=TRUE ("use temporary file?"), "error in"=w468, "variable name"=w461, "GOLPI ref. in"=w466) -> ("error out"=w467:errorcluster, "value"=w470:string, "GOLPI ref. out"=w465:T3)  [unwired: 5 in]
          n142 = Equal?(x=w460, y=w474) -> (x = y?=w464:bool)
          n143 = Equal?(x=w460, y=w470) -> (x = y?=w469:bool)
          n144 = And(x=w464, y=w469) -> (x .and. y?=w463:bool)
        }
        frame 18 {
          n145 = call-poly "Set Variable.vi"("use temporary file? (F)"=FALSE ("use temporary file? 2"), "error in"=w502, "value"=w479, "variable name"=w487, "GOLPI ref. in"=w501) -> ("error out"=w503:errorcluster, "GOLPI ref. out"=w500:T3)  [unwired: 5 in]
          n146 = call-poly "Get Variable.vi"("use temporary file? (F)"=FALSE ("use temporary file?"), "error in"=w503, "variable name"=w487, "GOLPI ref. in"=w500) -> ("error out"=w490:errorcluster, "value"=w499:string[], "GOLPI ref. out"=w491:T3)  [unwired: 5 in]
          n147 = call-poly "Get Variable.vi"("use temporary file? (F)"=TRUE ("use temporary file?"), "error in"=w490, "variable name"=w487, "GOLPI ref. in"=w491) -> ("error out"=w489:errorcluster, "value"=w482:string[], "GOLPI ref. out"=w488:T3)  [unwired: 5 in]
          n148 = Equal?(x=w479, y=w499) -> (x = y?=w493:bool[])
          n149 = Equal?(x=w479, y=w482) -> (x = y?=w486:bool[])
          n150 = And Array Elements(Boolean array=w493) -> (logical AND=w496:bool)
          n151 = Empty Array?(array=w493) -> (empty?=w494:bool)
          n152 = And Array Elements(Boolean array=w486) -> (logical AND=w483:bool)
          n153 = Empty Array?(array=w486) -> (empty?=w485:bool)
          n154 = Not(x=w494) -> (.not. x?=w495:bool)
          n155 = Not(x=w485) -> (.not. x?=w484:bool)
          n156 = Compound Arithmetic op=AND(w496, w495, w483, w484) -> (w492:bool)
        }
        frame 19 {
          n157 = call-poly "Set Variable.vi"("use temporary file? (F)"=TRUE ("use temporary file? 2"), "error in"=w527, "value"=w504, "variable name"=w509, "GOLPI ref. in"=w526) -> ("error out"=w528:errorcluster, "GOLPI ref. out"=w525:T3)  [unwired: 5 in]
          n158 = call-poly "Get Variable.vi"("use temporary file? (F)"=FALSE ("use temporary file?"), "error in"=w528, "variable name"=w509, "GOLPI ref. in"=w525) -> ("error out"=w511:errorcluster, "value"=w524:string[], "GOLPI ref. out"=w513:T3)  [unwired: 5 in]
          n159 = call-poly "Get Variable.vi"("use temporary file? (F)"=TRUE ("use temporary file?"), "error in"=w511, "variable name"=w509, "GOLPI ref. in"=w513) -> ("error out"=w510:errorcluster, "value"=w505:string[], "GOLPI ref. out"=w512:T3)  [unwired: 5 in]
          n160 = Equal?(x=w504, y=w524) -> (x = y?=w518:bool[])
          n161 = Equal?(x=w504, y=w505) -> (x = y?=w514:bool[])
          n162 = And Array Elements(Boolean array=w518) -> (logical AND=w521:bool)
          n163 = Empty Array?(array=w518) -> (empty?=w519:bool)
          n164 = And Array Elements(Boolean array=w514) -> (logical AND=w508:bool)
          n165 = Empty Array?(array=w514) -> (empty?=w515:bool)
          n166 = Not(x=w519) -> (.not. x?=w520:bool)
          n167 = Not(x=w515) -> (.not. x?=w507:bool)
          n168 = Compound Arithmetic op=AND(w521, w520, w508, w507) -> (w517:bool)
        }
        frame 20 {
          n169 = case shown="False" w529 {
            tunnel: w535 -> [w553 w557]
            tunnel: w534 -> [w552 w558]
            tunnel: [w547 w557] -> w533
            tunnel: [w545 TRUE] -> w532
            tunnel: [w537 w558] -> w531
            tunnel: ["test read to settle" ("variable name") "test read to settle - SKIPPED" ("variable name")] -> w530
            frame False {
              # "should generate\nnot supporte\nerror"
              n170 = call "Write Command.vi"("error in"=w552, "command"="for i=[1:10]\n   pause(1)\n   disp(i)\nend", "GOLPI ref. in"=w553) -> ("error out"=w550:errorcluster, "GOLPI ref. out"=w551:T3)  [unwired: 7 in]
              n171 = call "Read Output Till Settle.vi"("timeout [ms]"=u32 13000, "error in"=w550, "settled for [ms]"=u32 1100, "GOLPI ref. in"=w551) -> ("error out"=w538:errorcluster, "GOLPI ref. out"=w547:T3)  [unwired: 4 in, 2 out]
              n172 = Unbundle By Name(w538) -> ("code"=w542:i32)
              n173 = call "Generate Custom Error.vi"("GOLPI error"=Custom_Error_Codes_Enum_Type_Def.vi."90 Not supported in Matlab mode") -> ("error out"=w544:errorcluster)  [unwired: 10 in]
              n174 = Unbundle By Name(w544) -> ("code"=w543:i32)
              n175 = Not Equal?(x=w542, y=w543) -> (x != y?=w540:bool)
              n176 = Select(t=w538, s=w540, f=errorcluster {"status"=FALSE, "code"=0, "source"=""}) -> (s? t:f=w537:errorcluster)
              n177 = Unbundle By Name(w537) -> ("status"=w546:bool)
              n178 = Not(x=w546) -> (.not. x?=w545:bool)
            }
            frame True {
            }
          }
        }
        frame 21 {
          n179 = case shown="False" w559 {
            tunnel: w565 -> [w583 w587]
            tunnel: w564 -> [w582 w588]
            tunnel: ["test read to keyword" ("variable name") "test read to keyword - SKIPPED" ("variable name")] -> w563
            tunnel: [w578 w587] -> w562
            tunnel: [w574 TRUE] -> w561
            tunnel: [w566 w588] -> w560
            frame False {
              # "should generate\nnot supporte\nerror"
              n180 = call "Write Command.vi"("error in"=w582, "command"="for i=[1:10]\n   pause(1)\n  end\ndisp('testkeyword')", "GOLPI ref. in"=w583) -> ("error out"=w580:errorcluster, "GOLPI ref. out"=w579:T3)  [unwired: 7 in]
              n181 = call "Read Output Till Keyword.vi"("timeout [ms]"=u32 13000, "error in"=w580, "keywords"=string[] ["error", "testkeyword"], "GOLPI ref. in"=w579) -> ("error out"=w567:errorcluster, "GOLPI ref. out"=w578:T3)  [unwired: 4 in, 2 out]
              n182 = Unbundle By Name(w567) -> ("code"=w571:i32)
              n183 = call "Generate Custom Error.vi"("GOLPI error"=Custom_Error_Codes_Enum_Type_Def.vi."90 Not supported in Matlab mode") -> ("error out"=w573:errorcluster)  [unwired: 10 in]
              n184 = Unbundle By Name(w573) -> ("code"=w572:i32)
              n185 = Not Equal?(x=w571, y=w572) -> (x != y?=w569:bool)
              n186 = Select(t=w567, s=w569, f=errorcluster {"status"=FALSE, "code"=0, "source"=""}) -> (s? t:f=w566:errorcluster)
              n187 = Unbundle By Name(w566) -> ("status"=w575:bool)
              n188 = Not(x=w575) -> (.not. x?=w574:bool)
            }
            frame True {
            }
          }
        }
        frame 24 {
          # "should generate\nnot supporte\nerror"
          n189 = call "GOLPI full test - part structure.vi"("error in"=w601, "GOLPI ref. in"=w600) -> ("error out"=w594:errorcluster, "match"=w590:bool, "GOLPI ref. out"=w599:T3)  [unwired: 7 in]
          n190 = Unbundle By Name(w594) -> ("code"=w595:i32)
          n191 = call "Generate Custom Error.vi"("GOLPI error"=Custom_Error_Codes_Enum_Type_Def.vi."90 Not supported in Matlab mode") -> ("error out"=w597:errorcluster)  [unwired: 10 in]
          n192 = Unbundle By Name(w597) -> ("code"=w596:i32)
          n193 = Not Equal?(x=w595, y=w596) -> (x != y?=w589:bool)
          n194 = Compound Arithmetic op=OR(w590, invert w589) -> (w591:bool)
          n195 = Select(t=w594, s=w589, f=errorcluster {"status"=FALSE, "code"=0, "source"=""}) -> (s? t:f=w593:errorcluster)
        }
      }
      n196 = Concatenate Strings(w91, ": " ("string"), w93) -> (w92:string)
      n197 = Bundle("test result"=w116, w92) -> (w88:cluster{"test result":bool, string})  [unwired: 1 in]
      n198 = call "Write Command.vi"("error in"=w113, "command"="clear all", "GOLPI ref. in"=w115) -> ("error out"=w112:errorcluster, "GOLPI ref. out"=w114:T3)  [unwired: 7 in]
      n199 = Build Array (concatenate)(w87, w88) -> (w81:cluster{"test result":bool, string}[])
      n200 = property on="test results" class="Arr (strict)"("Value"=w81) -> ("Number of Rows"=w83:u32)  [unwired: 2 in, 2 out]
      n201 = Array Size(array=w81) -> (size(s)=w82:i32)
      n202 = Subtract(x=w82, y=w83) -> (x-y=w84:u32)
      n203 = expression code="max(i,0)"(w84) -> (w85:u32)
      n204 = Build Array(w85) -> (w86:u32[])
      n205 = property on="test results" class="Arr (strict)"("Index Values"=w86) -> ()  [unwired: 2 in, 2 out]
    }
  }
  "test results" <- w30
  n206 = Merge Errors(w44) -> (w22:errorcluster)
  n207 = And Array Elements(Boolean array=w48) -> (logical AND=w19:bool)
  "all tests result" <- w19
  n208 = invoke on="bitstream" class="DigNum (strict)" method="Reinit To Default"() -> (error out=w8:errorcluster)  [unwired: 3 in, 2 out]
  n209 = invoke on="console (write)" class="DigNum (strict)" method="Reinit To Default"() -> (error out=w3:errorcluster)  [unwired: 3 in, 2 out]
  n210 = Index Array(array=w15) -> (element=→"file":dbl)  [unwired: 1 in]
  n211 = Index Array(array=w13) -> (element #1=→"console":dbl, element #2=→"bitstream":dbl, element #3=→"pipe":dbl)  [unwired: 3 in]
  n212 = Index Array(array=w6) -> (element #1=→"console (write)":dbl, element #2=→"file (write)":dbl, element #3=→"pipe (write)":dbl)  [unwired: 3 in]
  n213 = Select(t=u32 6618880 ("Text.Text Colors:Text Color"), s=w19, f=u32 16711680 ("Text.Text Colors:Text Color")) -> (s? t:f=w17:u32)
  n214 = invoke on="console" class="DigNum (strict)" method="Reinit To Default"(error in=w8) -> (error out=w9:errorcluster)  [unwired: 2 in, 2 out]
  n215 = invoke on="pipe (write)" class="DigNum (strict)" method="Reinit To Default"(error in=w3) -> (error out=w1:errorcluster)  [unwired: 2 in, 2 out]
  n216 = call <vilib>:"Clear Errors.vi"("error in (no error)"=w22) -> ("error out"=w23:errorcluster)  [unwired: 5 in, 1 out]
  n217 = local read "wait for exit\n(press this again to exit)"() -> (w33:bool)
  n218 = property on="State" class="Str"(error in=w23, "Value"="ALL DONE!" ("State"), "Text.TextColor"=w17, "Text.BGColor"=u32 0 ("Text.Text Colors:BG Color")) -> ()  [unwired: 1 in, 2 out]
  n219 = invoke on="file" class="DigNum (strict)" method="Reinit To Default"(error in=w9) -> (error out=w7:errorcluster)  [unwired: 2 in, 2 out]
  n220 = invoke on="file (write)" class="DigNum (strict)" method="Reinit To Default"(error in=w1) -> ()  [unwired: 2 in, 3 out]
  n221 = invoke on="pipe" class="DigNum (strict)" method="Reinit To Default"(error in=w7) -> ()  [unwired: 2 in, 3 out]
  n222 = case shown="True" w33 {
    tunnel: [w603 w604] -> w34
    tunnel: w22 -> [w603 w604]
    frame False {
    }
    frame True {
      n223 = while {
        stop <- "wait for exit\n(press this again to exit)" continue-if-true
      }
    }
  }
  n224 = call "Quit GNU Octave.vi"("error in"=w34, "GOLPI ref. in"=w43) -> ("error out"=→"error out":errorcluster, "exit code"=→"exit code":i32)  [unwired: 8 in]
